vi "ObtainCanvas2D.vi"(10 "Name":string) -> (3 "Refnum out":refnum<k21>)   [LabVIEW 2013]
uses:
  <resource>/objmgr/Canvas2D.rc
panel:
  in  "Refnum out 2":refnum<k21>
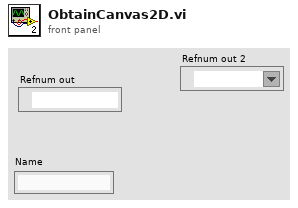
[diagram p1: front panel]
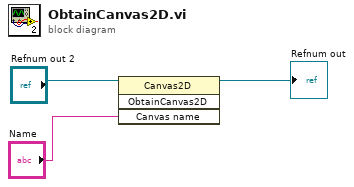
[diagram p0: block diagram]
diagram:
  n1 = invoke class="Canvas2D" method="ObtainCanvas2D"(reference="Refnum out 2", "Canvas name"="Name") -> (reference out=→"Refnum out":refnum<k21>)  [unwired: 2 in, 3 out]
